vi "ma_One-sided FFT Spectrum.vi"(8 "error in":errorcluster, 10 "dt":dbl format="%0.2f", 11 "signal (V)":dbl[](array[numeric]) format="%0.2f") -> (0 "error out":errorcluster, 2 "df":dbl format="%0.2f", 3 "FFT spectrum (Vrms)":cdb[](array[numeric]) format="%0.2f")   [LabVIEW 2020, in "NI_MAPro.lvlib"]
uses:
  NI_MAPro.lvlib
  NI_AALPro.lvlib
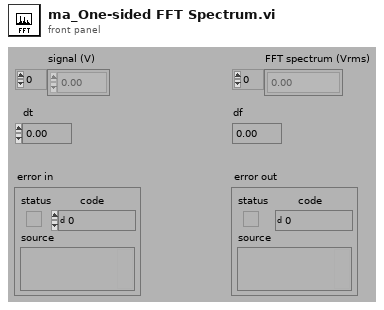
[diagram p1: front panel]
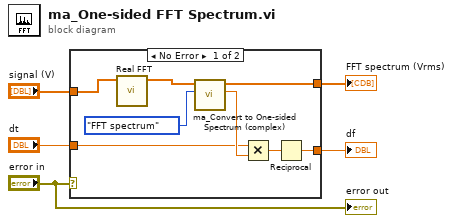
[diagram p0: block diagram]
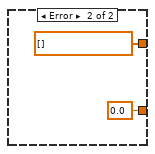
[diagram p2: hidden frame]
diagram:
  n1 = case shown="No Error" "error in" {
    tunnel: "signal (V)" -> [w13 _]
    tunnel: [w11 cdb[] [] ("one-sided spectrum (complex)")] -> w4
    tunnel: "dt" -> [w8 _]
    tunnel: [w7 0.0] -> w2
    frame No Error {
      n2 = call "Real FFT.vi"("X"=w13) -> ("FFT {X}"=w12:cdb[])  [unwired: 9 in, 1 out]
      n3 = call "ma_Convert to One-sided Spectrum (complex).vi"("spectrum type"=enum16{"FFT spectrum", "cross spectrum"}."FFT spectrum", "two-sided spectrum (complex)"=w12) -> ("block size"=w10:dbl, "one-sided spectrum (complex)"=w11:cdb[])  [unwired: 8 out]
      n4 = Multiply(x=w8, y=w10) -> (x*y=w9:dbl)
      n5 = Reciprocal(x=w9) -> (1/x=w7:dbl)
    }
    frame Error {
    }
  }
  "df" <- w2
  "FFT spectrum (Vrms)" <- w4
  "error out" <- "error in"
